vi "GSI-HVSwitch2.get address.vi"(0 "i ref in":refnum<vi>, 5 "error in (no error)":errorcluster) -> (14 "i ref out":refnum<vi>, 16 "SDEX address":T1={"VISA resource name"="", "HEX address"=0, "VISA Timeout Value (1000 ms)"=1000, "Lock Timeout (1000 ms)"=1000, "semaphore"=refnum, "Baud rate"=0, "revision"=enum."unknown", "deviceInfo"=""} {"HEX address" format="%.0x"}, 19 "error out":errorcluster)   [LabVIEW 2014, in "GSI-HVSwitch2.lvlib"]
doc: "Gets the SDEX cluster containing the VISA resource etc."
uses:
  GSI-HVSwitch2.lvlib
  instr.lib/SDEX/SDEX.VISA Control.ctl
  instr.lib/SDEX/SDEX.revisionType.ctl
  instr.lib/SDEX/SDEXDriver.lvlib
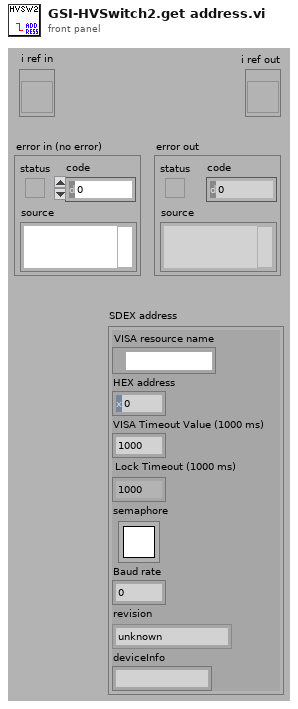
[diagram p1: front panel]
types:
  T1 = typedef "SDEXDriver.lvlib/SDEX.VISA Control.ctl" = cluster{"VISA resource name":refnum<visa-resource-name>, "HEX address":u16, "VISA Timeout Value (1000 ms)":u32, "Lock Timeout (1000 ms)":u32, "semaphore":T2, "Baud rate":u32, "revision":T3, "deviceInfo":string}
  T2 = typedef "Semaphore RefNum" = refnum<k1>
  T3 = typedef "SDEXDriver.lvlib/SDEX.revisionType.ctl" = enum16{"unknown", "hvamp3", "hvswi1", "htrp0", "WDG0"}
  T4 = typedef "GSI-HVSwitch2.lvlib/GSI-HVSwitch2.i attribute.ctl" = cluster{"SDEX VISA Cluster":T1, "SetVoltage SW0":dbl, "SetVoltage SW1":dbl, "ActTempAmp":dbl, "ActTempPS1":dbl, "ActTempPS2":dbl, "mode":T5, "interfaceInitialized":bool, "serviceIDs":cluster{"nomVoltage0ID":i32, "nomVoltage1ID":i32, "actTempAmpID":i32, "actTempPS1ID":i32, "actTempPS2ID":i32, "modeID":i32}, "usedChannels":i32}
  T5 = typedef "GSI-HVSwitch2.lvlib/GSI-HVSwitch2.mode.ctl" = enum16{"unknown", "switch", "stepper"}
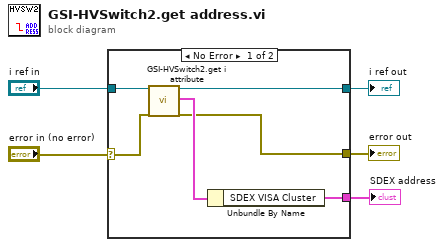
[diagram p0: block diagram]
diagram:
  n1 = case shown="No Error" "error in (no error)" {
    selector: "error in (no error)" -> [w6 w12]
    tunnel: "i ref in" -> [w11 w13]
    tunnel: [w9 w13] -> w4
    tunnel: [w8 w12] -> w3
    tunnel: [w7 _] -> w2
    frame No Error {
      n2 = call "GSI-HVSwitch2.get i attribute.vi"("i ref in"=w11, "error in (no error)"=w6) -> ("i ref out"=w9:refnum<vi>, "i attribute"=w10:T4, "error out"=w8:errorcluster)  [unwired: 15 in]
      n3 = Unbundle By Name(w10) -> ("SDEX VISA Cluster"=w7:T1)
    }
    frame Error {
    }
  }
  "error out" <- w3
  "i ref out" <- w4
  "SDEX address" <- w2
